vi "Read Node Controller.vi"(8 "error in (no error)":errorcluster, 11 "Superior Actor in":refnum<class "Root Actor.lvclass">) -> (0 "error out":errorcluster, 2 "Node Controller":refnum<class "Node Controller.lvclass">, 3 "Superior Actor out":refnum<class "Root Actor.lvclass">)   [LabVIEW 2024, in "Root Actor.lvclass"]
uses:
  Root Actor.lvclass
  Actor Assistant/Root Actor Node Controller/Node Controller.lvclass
  Root Actor.lvclass/Root Actor.ctl
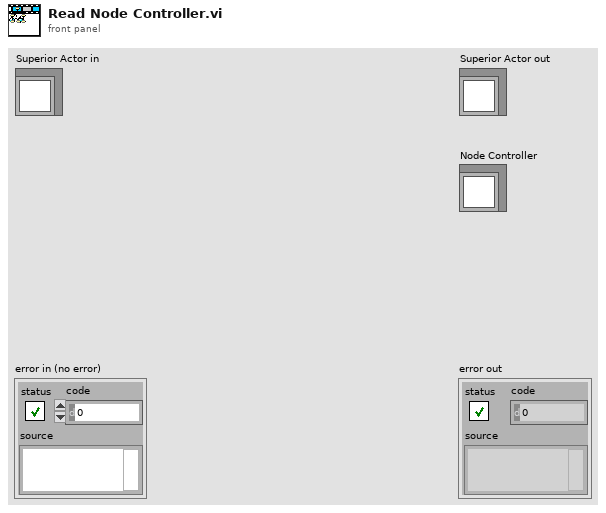
[diagram p1: front panel]
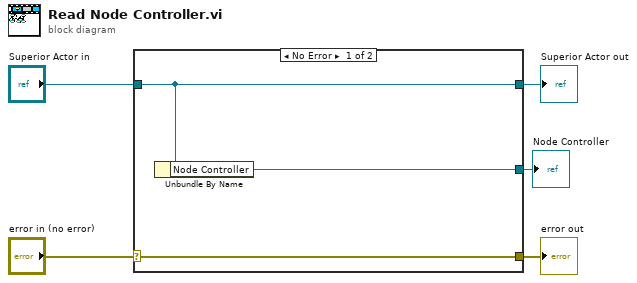
[diagram p0: block diagram]
diagram:
  n1 = case shown="No Error" "error in (no error)" {
    selector: "error in (no error)" -> [w8 w9]
    tunnel: [w8 w9] -> w4
    tunnel: [w7 w10] -> w2
    tunnel: "Superior Actor in" -> [w7 w10]
    tunnel: [w6 _] -> w1
    frame No Error {
      n2 = Unbundle By Name(w7) -> ("Node Controller"=w6:refnum<class "Node Controller.lvclass">)
    }
    frame Error {
    }
  }
  "error out" <- w4
  "Superior Actor out" <- w2
  "Node Controller" <- w1
